vi "Add Widget to Container.vi"(5 "Container":refnum<class "QWidget.lvclass">, 8 "Error In":errorcluster, 9 "Label":string, 10 "Widget":refnum<class "QWidget.lvclass">, 11 "Tool Box Builder in":refnum<class "Tool Box Builder.lvclass">) -> (0 "Error Out":errorcluster, 3 "Tool Box Builder out":refnum<class "Tool Box Builder.lvclass">)   [LabVIEW 2014, in "Dynamic GUI Composition and Management.lvlib" / "Tool Box Builder.lvclass"]
doc: "Copyright (c) 2016 Sze Howe Koh\nThis code is licensed under the MIT license"
uses:
  Tool Box Builder.lvclass
  src/LabVIEW/Qt Widgets/QWidget/QWidget.lvclass
  src/LabVIEW/Qt Widgets/QToolBox/QToolBox.lvclass
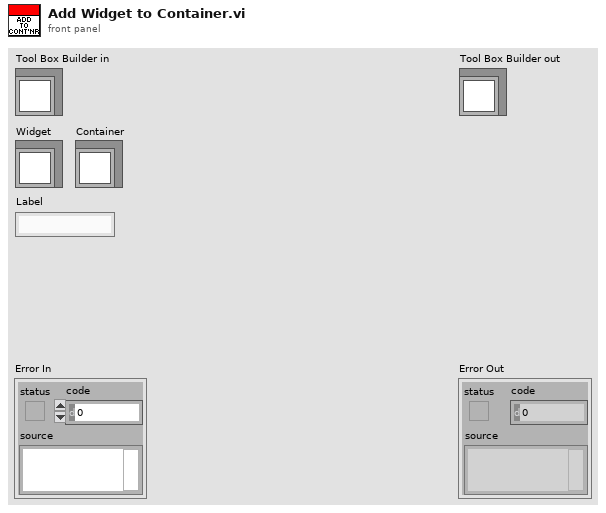
[diagram p1: front panel]
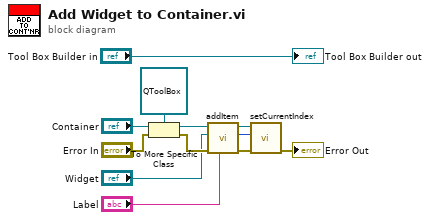
[diagram p0: block diagram]
diagram:
  n1 = To More Specific Class(target class=refnum<class "QToolBox.lvclass"> refnum ("QToolBox In"), reference="Container", error in="Error In") -> (specific class reference=w5:refnum<class "QToolBox.lvclass">, error out=w8:errorcluster)
  n2 = call "addItem.vi"("text"="Label", "Error In"=w8, "widget"="Widget", "QToolBox In"=w5) -> ("Error Out"=w2:errorcluster, "Value"=w3:i32, "QToolBox Out"=w4:refnum<class "QToolBox.lvclass">)  [unwired: 5 in]
  n3 = call "setCurrentIndex.vi"("Error In"=w2, "index"=w3, "QToolBox In"=w4) -> ("Error Out"=→"Error Out":errorcluster)  [unwired: 7 in, 1 out]
  "Tool Box Builder out" <- "Tool Box Builder in"
